vi "RT Loop - System Health and Monitoring.vi"(11 "Message Queue":refnum<queue>) -> ()   [LabVIEW 2017]
uses:
  support/Message Queue/Message Cluster.ctl
  controls/Control State.ctl
  Globals/Global - Configuration Options.vi
  <vilib>/nisyscfg/Close (System).vi
  <vilib>/NI_Real-Time Target Support.lvlib
  <vilib>/nisyscfg/nisyscfg.lvlib
  <resource>/objmgr/nisysapi.rc
  <vilib>/Utility/RT CPU Load.ctl
  support/Message Queue/Message Queue.lvlib
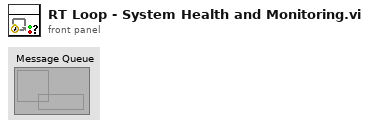
[diagram p1: front panel]
types:
  T1 = typedef "NI_Real-Time Target Support.lvlib/RT CPU Load.ctl" = cluster{"Total (%)":dbl, "Time Critical (%)":dbl, "Timed Structures (%)":dbl, "High (%)":dbl, "Above Normal (%)":dbl, "Normal (%)":dbl, "Background (%)":dbl, "Idle (%)":dbl, "ISR (%)":dbl}
  T2 = typedef "Control State.ctl" = enum16{"Safe State", "Control (PID)"}
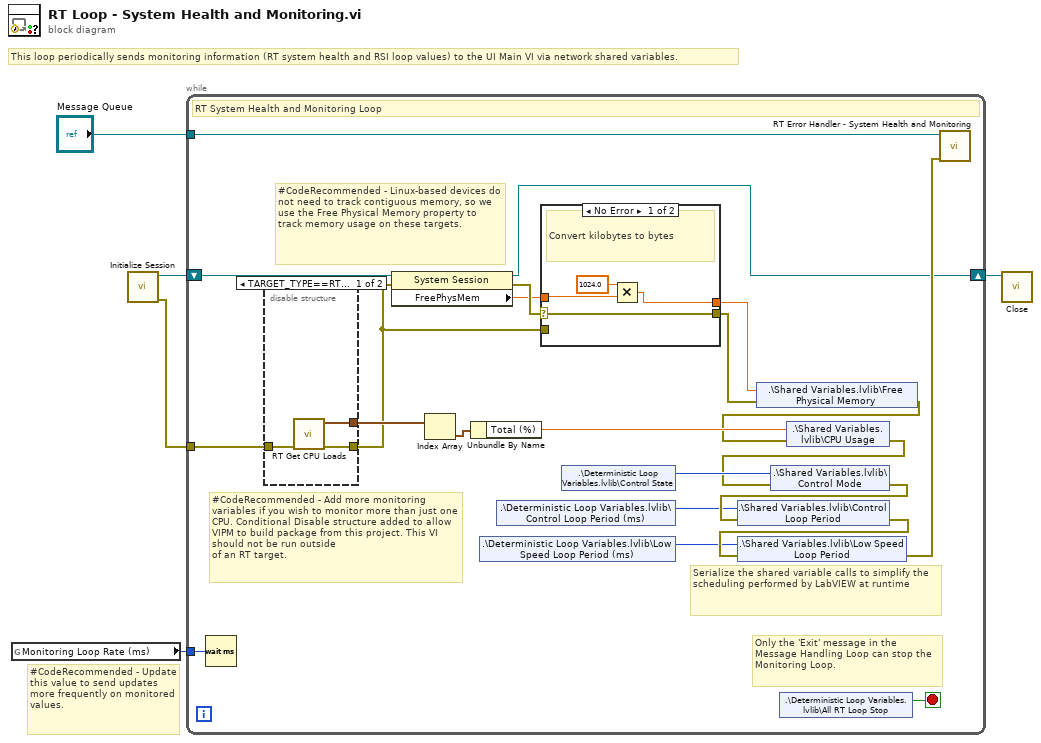
[diagram p0: block diagram]
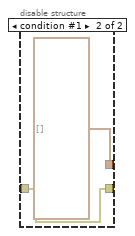
[diagram p2: hidden frame]
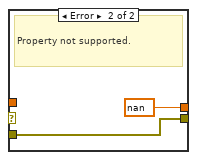
[diagram p3: hidden frame]
diagram:
  # "#CodeRecommended - Update this value to send updates more frequently on monitored values."
  # "This loop periodically sends monitoring information (RT system health and RSI loop values) to the UI Main VI via network shared variables."
  n1 = global read "Global - Configuration Options.vi" "Monitoring Loop Rate (ms)"() -> (w4:u32)
  n2 = call <vilib>:"Initialize Session.vi"() -> ("error out"=w1:errorcluster, "Session out"=w3:refnum<k21>)  [unwired: 10 in]
  n3 = while {
    tunnel: "Message Queue" -> [w24]
    tunnel: w4 -> [w23]
    shift-right: [w6] -> w2
    shift-left: w3 -> [w13]
    tunnel: w1 -> [w12]
    stop <- w19 stop-if-true
    # "#CodeRecommended - Add more monitoring variables if you wish to monitor more than just one CPU. Conditional Disable structure added to allow VIPM to build package from this project. This VI should not be run outside\nof an RT target."
    # "#CodeRecommended - Linux-based devices do not need to track contiguous memory, so we use the Free Physical Memory property to track memory usage on these targets."
    # "Serialize the shared variable calls to simplify the scheduling performed by LabVIEW at runtime"
    # "Only the 'Exit' message in the  Message Handling Loop can stop the Monitoring Loop."
    # "RT System Health and Monitoring Loop"
    n4 = Wait (ms)(milliseconds to wait=w23) -> ()  [unwired: 1 out]
    n5 = disable-structure shown="TARGET_TYPE==RT, Default" {
      disable-tunnel: [w30 T1[] [] ("CPU loads")] -> w27
      disable-tunnel: w12 -> [w29 w31]
      disable-tunnel: [w28 w31] -> w9
      frame condition #0 (active) {
        n6 = call <vilib>:"RT Get CPU Loads.vi"("error in (no error)"=w29) -> ("error out"=w28:errorcluster, "CPU loads"=w30:T1[])  [unwired: 9 in]
      }
      frame condition #1 {
      }
    }
    n7 = property class="System Session"(reference=w13, error in=w9) -> (reference out=w6:refnum<k21>, error out=w11:errorcluster, "FreePhysMem"=w10:dbl)
    n8 = Index Array(array=w27) -> (element=w26:T1)  [unwired: 1 in]
    n9 = Unbundle By Name(w26) -> ("Total (%)"=w25:dbl)
    n10 = shared-variable ".\\Deterministic Loop Variables.lvlib\\Low Speed Loop Period (ms)"() -> (w16:u32)  [unwired: 1 in, 1 out]
    n11 = shared-variable ".\\Deterministic Loop Variables.lvlib\\Control Loop Period (ms)"() -> (w17:u32)  [unwired: 1 in, 1 out]
    n12 = case shown="No Error" w11 {
      selector: w11 -> [w33 _]
      tunnel: w10 -> [w35 _]
      tunnel: [w34 nan] -> w8
      tunnel: [w33 w37] -> w7
      tunnel: w9 -> [_ w37]
      frame No Error {
        # "Convert kilobytes to bytes"
        n13 = Multiply(x=1024.0, y=w35) -> (x*y=w34:dbl)
      }
      frame Error {
        # "Property not supported."
      }
    }
    n14 = shared-variable ".\\Deterministic Loop Variables.lvlib\\Control State"() -> (w18:T2)  [unwired: 1 in, 1 out]
    n15 = shared-variable ".\\Shared Variables.lvlib\\Free Physical Memory"(w8, error in=w7) -> (error out=w15:errorcluster)
    n16 = shared-variable ".\\Deterministic Loop Variables.lvlib\\All RT Loop Stop"() -> (w19:bool)  [unwired: 1 in, 1 out]
    n17 = shared-variable ".\\Shared Variables.lvlib\\CPU Usage"(w25, error in=w15) -> (error out=w14:errorcluster)
    n18 = shared-variable ".\\Shared Variables.lvlib\\Control Mode"(w18, error in=w14) -> (error out=w20:errorcluster)
    n19 = shared-variable ".\\Shared Variables.lvlib\\Control Loop Period"(w17, error in=w20) -> (error out=w22:errorcluster)
    n20 = shared-variable ".\\Shared Variables.lvlib\\Low Speed Loop Period"(w16, error in=w22) -> (error out=w21:errorcluster)
    n21 = call "RT Error Handler - System Health and Monitoring.vi"("error in (no error)"=w21, "Message Queue"=w24) -> ()  [unwired: 9 in, 1 out]
  }
  n22 = call-poly <vilib>:"Close.vi"("Session in"=w2) -> ()  [unwired: 10 in, 1 out]
